vi "List Databases.vi"(8 "error in (no error)":errorcluster, 10 "Context":string, 11 "sqlite in":refnum<class "sqlite3.lvclass">) -> (0 "error out":errorcluster, 2 "databases":string[](array[string]), 3 "sqlite out":refnum<class "sqlite3.lvclass">)   [LabVIEW 2020, in "sqlite3.lvlib" / "sqlite3.lvclass"]
uses:
  sqlite3.lvclass
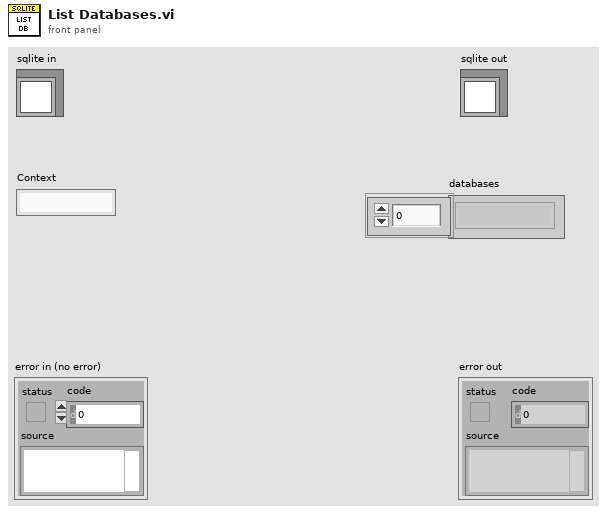
[diagram p1: front panel]
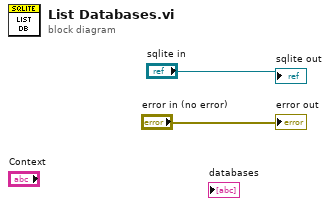
[diagram p0: block diagram]
diagram:
  "error out" <- "error in (no error)"
  "sqlite out" <- "sqlite in"
